vi "Choreo_Util_AllianceFlipRotation2d.vi"(11 "Rotation":T1={"VALUE"=0.0, "COS"=1.0, "SIN"=0.0} {"SIN" format="%13.4f"; "COS" format="%13.4f"; "VALUE" format="%13.4f"}) -> (3 "FlippedRotation":T1={"VALUE"=0.0, "COS"=1.0, "SIN"=0.0} {"SIN" format="%13.4f"; "COS" format="%13.4f"; "VALUE" format="%13.4f"})   [LabVIEW 2019, in "ChoreoLib.lvlib"]
doc: "trajectory, mirrored across the field midline.\n\nInputs: \n - ChoreoTrajectory - cluster - Input trajectory\n\nOutputs:\n - Flipped Trajectory - cluster - trajectory, mirrored across the field midline."
uses:
  ChoreoLib.lvlib
  Choreo_Choreo_Globals.vi
  <vilib>/Rock Robotics/WPI/ThirdParty/JAS_Junk/TrajLib/Trajectory_Library.lvlib
  <vilib>/Rock Robotics/WPI/ThirdParty/JAS_Junk/TrajLib/TypeDef/ROTATION2D.ctl
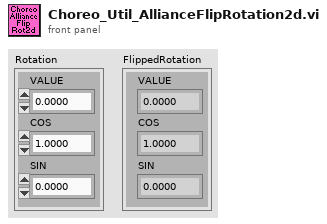
[diagram p1: front panel]
types:
  T1 = typedef "Trajectory_Library.lvlib/ROTATION2D.ctl" = cluster{"VALUE":dbl, "COS":dbl, "SIN":dbl}
  T2 = typedef "ChoreoLib.lvlib/Choreo_Util_AllianceFlipType.ctl" = enum16{"MIRRORED", "ROTATE_AROUND"}
  T3 = cluster{"Year":i32, "AllianceFlipType":T2, "FieldLength":dbl, "FieldWidth":dbl}
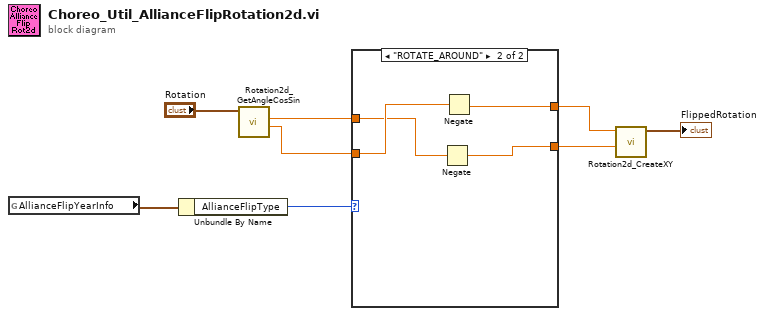
[diagram p0: block diagram]
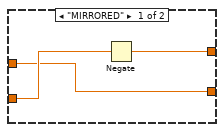
[diagram p2: hidden frame]
diagram:
  n1 = global read "Choreo_Choreo_Globals.vi" "AllianceFlipYearInfo"() -> (w8:T3)
  n2 = Unbundle By Name(w8) -> ("AllianceFlipType"=w7:T2)
  n3 = call <vilib>:"Rotation2d_GetAngleCosSin.vi"("in ROTATION"="Rotation") -> ("Cosine"=w4:dbl, "Sine"=w1:dbl)  [unwired: 8 in, 1 out]
  n4 = case shown="\"ROTATE_AROUND\"" w7 {
    tunnel: w4 -> [w11 w15]
    tunnel: [w10 w14] -> w3
    tunnel: [w9 w12] -> w2
    tunnel: w1 -> [w9 w13]
    frame "MIRRORED" {
      n5 = Negate(x=w11) -> (-x=w10:dbl)
    }
    frame "ROTATE_AROUND" {
      n6 = Negate(x=w13) -> (-x=w12:dbl)
      n7 = Negate(x=w15) -> (-x=w14:dbl)
    }
  }
  n8 = call <vilib>:"Rotation2d_CreateXY.vi"("Y or sine"=w2, "X or  cosine"=w3) -> ("ROTATION"=→"FlippedRotation":T1)  [unwired: 9 in]
